vi "TCP Service.vi"() -> ()   [LabVIEW 2020, in "GenNet-Server.lvlib"]
doc: "____\nHAMPEL SOFTWARE ENGINEERING v3.8.0 (2023-12-18 14:41)"
uses:
  GenNet-Server.lvlib
  Stop Argument--cluster.ctl
  GenNet Protocols/GenNet Protocol.lvclass
panel:
  in  "GenNet Protocol":refnum<class "GenNet Protocol.lvclass">
  in  "Stop Module":refnum<user-event>
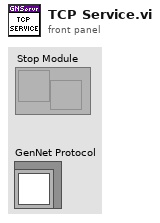
[diagram p1: front panel]
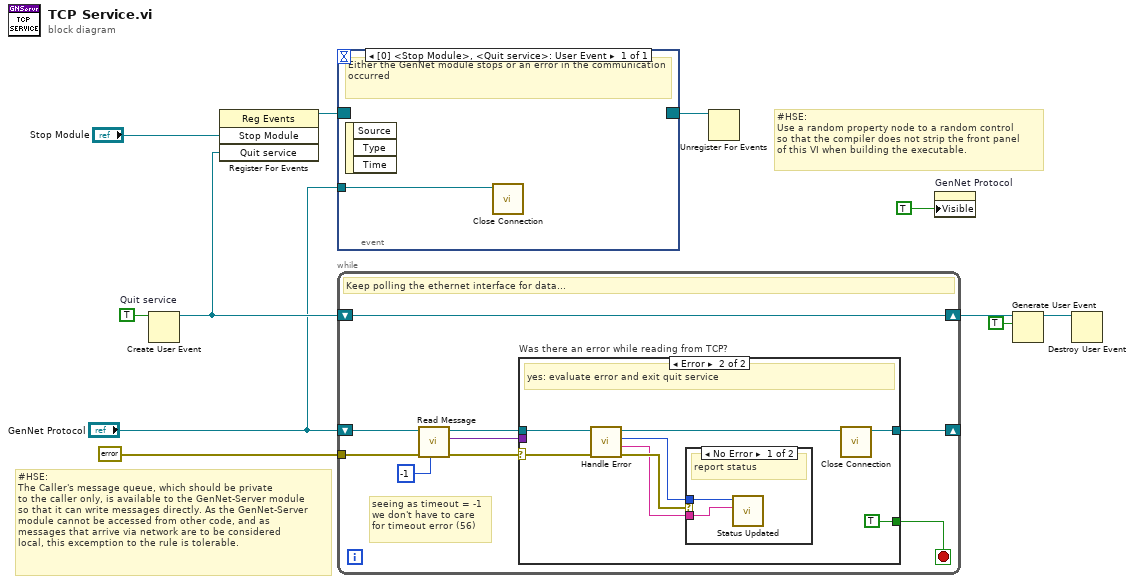
[diagram p0: block diagram]
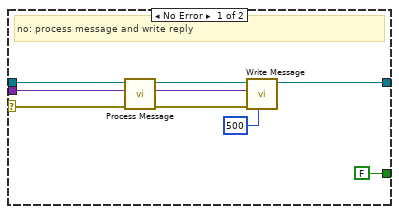
[diagram p2: hidden frame]
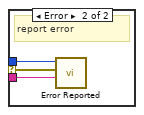
[diagram p3: hidden frame]
diagram:
  w9 = TRUE  # Quit service
  # "#HSE: \nUse a random property node to a random control \nso that the compiler does not strip the front panel \nof this VI when building the executable."
  # "#HSE: \nThe Caller's message queue, which should be private \nto the caller only, is available to the GenNet-Server module \nso that it can write messages directly. As the GenNet-Server\nmodule cannot be accessed from other code, and as \nmessages that arrive via network are to be considered \nlocal, this excemption to the rule is tolerable."
  n1 = Create User Event(user event datatype=w9) -> (user event=w8:refnum<user-event>)  [unwired: 1 in, 1 out]
  n2 = register-events("Stop Module", w8) -> (reference out=w10:refnum<event-registration>)  [unwired: 2 in, 1 out]
  n3 = event shown="[0] <Stop Module>, <Quit service>: User Event" {
    selector: w10 -> [_]
    dyn-events: [_] -> w4
    timeout: _ -> [_]
    tunnel: "GenNet Protocol" -> [w12]
    event User Event {
      # "Either the GenNet module stops or an error in the communication occurred"
      n4 = event-data() -> ()  [unwired: 1 in, 3 out]
      n5 = call-dynamic "Close Connection.vi"("GenNet Protocol in"=w12) -> ()  [unwired: 9 in, 2 out]
    }
  }
  n6 = while {
    shift-right: [w14] -> _
    shift-left: "GenNet Protocol" -> [w19]
    shift-right: [w21] -> w7
    shift-left: w8 -> [w21]
    tunnel: errorcluster {"status"=FALSE, "code"=0, "source"=""} ("error out") -> [w18]
    stop <- w20 stop-if-true
    # "seeing as timeout = -1\nwe don't have to care\nfor timeout error (56)"
    # "Keep polling the ethernet interface for data..."
    n7 = call-dynamic "Read Message.vi"("timeout ms (25000)"=-1, "error in (no error)"=w18, "GenNet Protocol in"=w19) -> ("error out"=w17:errorcluster, "Message"=w16:variant, "GenNet Protocol out"=w15:refnum<class "GenNet Protocol.lvclass">)  [unwired: 6 in]
    n8 = case "Was there an error while reading from TCP?" shown="Error" w17 {
      selector: w17 -> [w29 w37]
      tunnel: [FALSE TRUE] -> w20
      tunnel: w16 -> [w28 _]
      tunnel: w15 -> [w27 w36]
      tunnel: [w23 w31] -> w14
      frame No Error {
        # "no: process message and write reply"
        n9 = call-dynamic "Process Message.vi"("error in (no error)"=w29, "Request Message"=w28, "GenNet Protocol in"=w27) -> ("error out"=w26:errorcluster, "Reply Message"=w25:variant, "GenNet Protocol out"=w24:refnum<class "GenNet Protocol.lvclass">)  [unwired: 6 in]
        n10 = call-dynamic "Write Message.vi"("timeout ms (25000)"=500, "error in (no error)"=w26, "Message"=w25, "GenNet Protocol in"=w24) -> ("GenNet Protocol out"=w23:refnum<class "GenNet Protocol.lvclass">)  [unwired: 6 in, 1 out]
      }
      frame Error {
        # "yes: evaluate error and exit quit service"
        n11 = call-dynamic "Handle Error.vi"("error in (no error)"=w37, "GenNet Protocol in"=w36) -> ("error out"=w35:errorcluster, "Add Info for Error Broadcast"=w33:string, "Module ID for Error Broadcast"=w34:i32, "GenNet Protocol out"=w32:refnum<class "GenNet Protocol.lvclass">)  [unwired: 6 in]
        n12 = case shown="No Error" w35 {
          selector: w35 -> [_ w43]
          tunnel: w34 -> [w40 w42]
          tunnel: w33 -> [w39 w41]
          frame No Error {
            # "report status"
            n13 = call "Status Updated.vi"("Status"=w39, "Module ID"=w40) -> ()  [unwired: 9 in, 1 out]
          }
          frame Error {
            # "report error"
            n14 = call "Error Reported.vi"("Additional Information"=w41, "Error"=w43, "Module ID"=w42) -> ()  [unwired: 8 in, 1 out]
          }
        }
        n15 = call-dynamic "Close Connection.vi"("GenNet Protocol in"=w32) -> ("GenNet Protocol out"=w31:refnum<class "GenNet Protocol.lvclass">)  [unwired: 9 in, 1 out]
      }
    }
  }
  n16 = Unregister For Events(event registration refnum=w4) -> ()  [unwired: 1 in, 1 out]
  n17 = property on="GenNet Protocol" class="LVClassControl (strict)"("Visible"=TRUE) -> ()  [unwired: 2 in, 2 out]
  n18 = Generate User Event(user event=w7, event data cluster=TRUE ("event data")) -> (user event out=w5:refnum<user-event>)  [unwired: 2 in, 1 out]
  n19 = Destroy User Event(user event=w5) -> ()  [unwired: 1 in, 1 out]
